vi "Test Suite.Serialize - Invalid character in Name - XML does not contain invalid character.vi"() -> ()   [LabVIEW 2013, in "JUnit XML Tests.lvlib"]
uses:
  JUnit XML Tests.lvlib
  JUnit XML/Test Suite/Test Suite.lvclass/Test Suite.ctl
  JUnit XML/Test Suite/Write Timestamp.vi
  <vilib>/xml/Close Reference(Node).vi
  <vilib>/addons/_JKI Toolkits/Caraya/classes/Assert/Assert Equal Value_Variant.vi
  JUnit XML/JUnit XML.lvlib
  JUnit XML/Test Suite/Test Suite.lvclass
  <vilib>/addons/_JKI Toolkits/Caraya/classes/Test/Test.lvclass
  <vilib>/addons/_JKI Toolkits/Caraya/classes/Assert/Assert.lvclass
  <resource>/objmgr/DOMUserDefRef.rc
  <vilib>/xml/NI_XML.lvlib
panel:
  out "error out":errorcluster
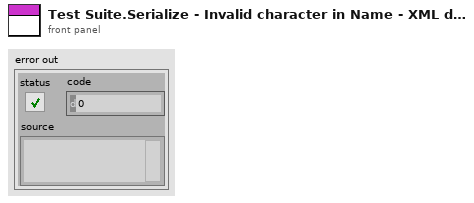
[diagram p1: front panel]
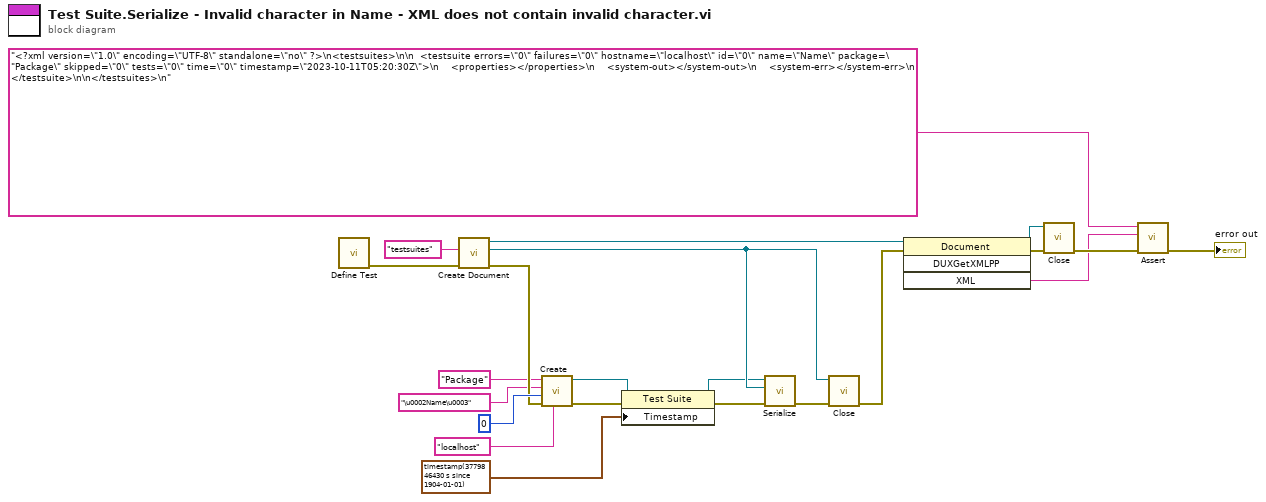
[diagram p0: block diagram]
diagram:
  n1 = call <vilib>:"Define Test.vi"() -> ("error out"=w22:errorcluster)  [unwired: 10 in, 1 out]
  n2 = call "Create Document.vi"("error in (no error)"=w22, "Root Element Name"="testsuites") -> ("error out"=w18:errorcluster, "Root Element"=w14:refnum<k20>, "Document"=w17:refnum<k20>)  [unwired: 7 in]
  n3 = call "Create.vi"("Hostname (\"localhost\")"="localhost" ("Package"), "error in (no error)"=w18, "Id"=0, "Name"="\u0002Name\u0003" ("Package"), "Package"="Package") -> ("error out"=w21:errorcluster, "Test Suite"=w3:refnum<class "Test Suite.lvclass">)  [unwired: 5 in]
  n4 = property class="Test Suite"(reference=w3, error in=w21, "Timestamp"=timestamp(3779846430.123 s since 1904-01-01)) -> (reference out=w2:refnum<class "Test Suite.lvclass">, error out=w4:errorcluster)
  n5 = call "Serialize.vi"("error in (no error)"=w4, "Element in"=w14, "Test Suite in"=w2) -> ("error out"=w16:errorcluster)  [unwired: 7 in, 1 out]
  n6 = call-poly <vilib>:"Close.vi"("error in (no error)"=w16, "node"=w14) -> ("error out"=w15:errorcluster)  [unwired: 7 in]
  n7 = invoke class="Document" method="DUXGetXMLPP"(reference=w17, error in=w15) -> (reference out=w12:refnum<k20>, error out=w13:errorcluster, "XML"=w10:string)  [unwired: 2 in, 1 out]
  n8 = call-poly <vilib>:"Close.vi"("error in (no error)"=w13, "node"=w12) -> ("error out"=w11:errorcluster)  [unwired: 7 in]
  n9 = call-poly <vilib>:"Assert.vi"("error in (no error)"=w11, "Actual"=w10, "Expected"="<?xml version=\"1.0\" encoding=\"UTF-8\" standalone=\"no\" ?>\n<testsuites>\n\n  <testsuite errors=\"0\" failures=\"0\" hostname=\"localhost\" id=\"0\" name=\"Name\" package=\"Package\" skipped=\"0\" tests=\"0\" time=\"0\" timestamp=\"2023-10-11T05:20:30Z\">\n    <properties></properties>\n    <system-out></system-out>\n    <system-err></system-err>\n  </testsuite>\n\n</testsuites>\n") -> ("error out"=→"error out":errorcluster)  [unwired: 7 in, 1 out]
